vi "Get ControlCANDLL Path.vi"(8 "error in (no error)":errorcluster caption="错误输入（无错误）") -> (0 "error out":errorcluster caption="错误输出", 3 "拆分的路径":path)   [LabVIEW 2020, in "ZLGCAN.lvclass"]
uses:
  ZLGCAN.lvclass
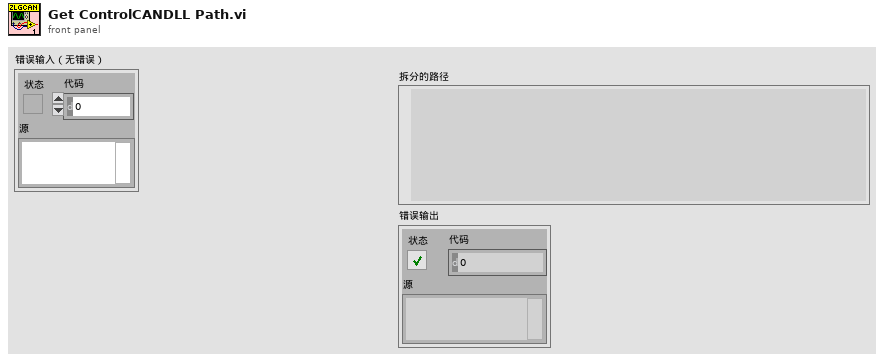
[diagram p1: front panel]
types:
  T1 = enum32{"invalid app kind", "Development System", "Run Time System", "Student Edition", "Embedded LabVIEW", "Evaluation", "Custom"}
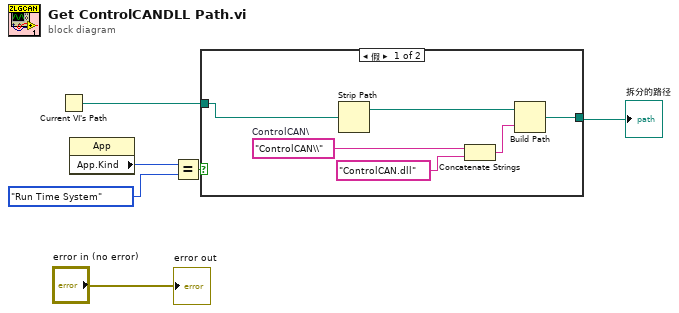
[diagram p0: block diagram]
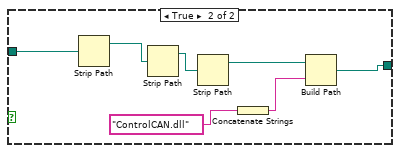
[diagram p2: hidden frame]
diagram:
  n1 = Current VI's Path() -> (path=w3:path)
  n2 = property class="App"() -> ("App.Kind"=w6:T1)  [unwired: 2 in, 2 out]
  n3 = Equal?(x=w6, y=T1."Run Time System" ("应用程序:类别")) -> (x = y?=w4:bool)
  n4 = case shown="假" w4 {
    tunnel: w3 -> [w12 w19]
    tunnel: [w7 w13] -> w1
    frame False {
      w11 = "ControlCAN\\"  # ControlCAN\
      n5 = Strip Path(path=w12) -> (stripped path=w9:path)  [unwired: 1 out]
      n6 = Concatenate Strings(w11, "ControlCAN.dll" ("字符串")) -> (w8:string)
      n7 = Build Path(base path=w9, name or relative path=w8) -> (appended path=w7:path)
    }
    frame True {
      n8 = Strip Path(path=w19) -> (stripped path=w18:path)  [unwired: 1 out]
      n9 = Strip Path(path=w18) -> (stripped path=w17:path)  [unwired: 1 out]
      n10 = Strip Path(path=w17) -> (stripped path=w16:path)  [unwired: 1 out]
      n11 = Concatenate Strings("ControlCAN.dll" ("字符串")) -> (w14:string)
      n12 = Build Path(base path=w16, name or relative path=w14) -> (appended path=w13:path)
    }
  }
  "拆分的路径" <- w1
  "error out" <- "error in (no error)"
